vi "string length fiinding 4.vi"() -> ()   [LabVIEW 2025]
panel:
  out "Numeric":dbl
  in  "String":string
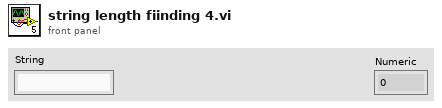
[diagram p1: front panel]
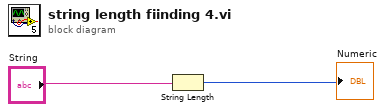
[diagram p0: block diagram]
diagram:
  n1 = String Length(string="String") -> (length=→"Numeric":i32)
